vi "De-Initialize.vi"(8 "error in (no error)":errorcluster, 11 "RFSoC Driver in":refnum<class "RFSoC Driver.lvclass">) -> (0 "error out":errorcluster, 3 "RFSoC Driver out":refnum<class "RFSoC Driver.lvclass">)   [LabVIEW 2020, in "RFSoC Driver.lvclass"]
uses:
  RFSoC Driver.lvclass
  RFSoC Driver.lvclass/RFSoC Driver.ctl
  Pulse Driver/Pulse Driver.lvclass
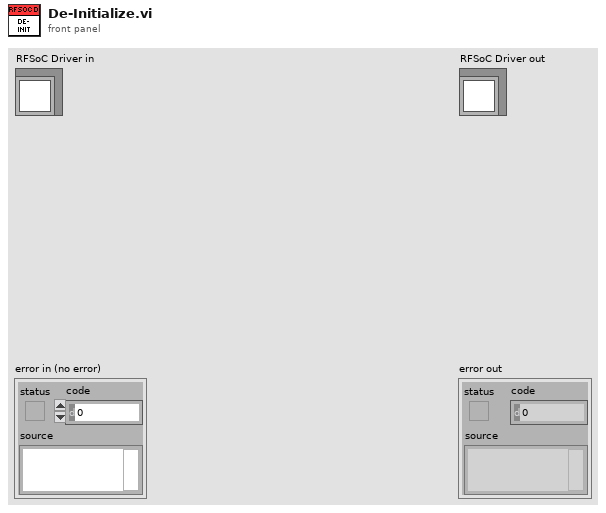
[diagram p1: front panel]
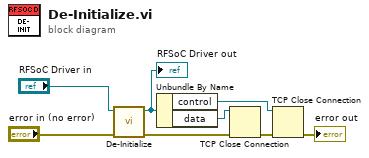
[diagram p0: block diagram]
diagram:
  n1 = call-parent "De-Initialize.vi"("error in (no error)"="error in (no error)", "Instrument Driver in"="RFSoC Driver in") -> ("error out"=w2:errorcluster, "Instrument Driver out"=w6:refnum<class "RFSoC Driver.lvclass">)  [unwired: 8 in]
  "RFSoC Driver out" <- w6
  n2 = Unbundle By Name(w6) -> ("control"=w5:refnum<k5>, "data"=w4:refnum<k5>)
  n3 = TCP Close Connection(connection ID=w4, error in (no error)=w2) -> (error out=w3:errorcluster)  [unwired: 1 in, 1 out]
  n4 = TCP Close Connection(connection ID=w5, error in (no error)=w3) -> (error out=→"error out":errorcluster)  [unwired: 1 in, 1 out]
